vi "WPI_ADI_IMU_ComplementaryFilter.vi"(7 "Filter Coefficient a":dbl, 8 "dt (ms)":dbl, 10 "Gyro (degrees/second)":dbl, 11 "Accelerometer (degrees)":dbl) -> (2 "timeConstant":dbl, 3 "Filtered":dbl)   [LabVIEW 2015, in "FRC ADI MXP IMU.lvlib"]
uses:
  FRC ADI MXP IMU.lvlib
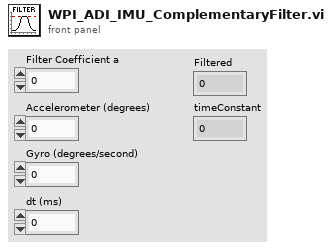
[diagram p1: front panel]
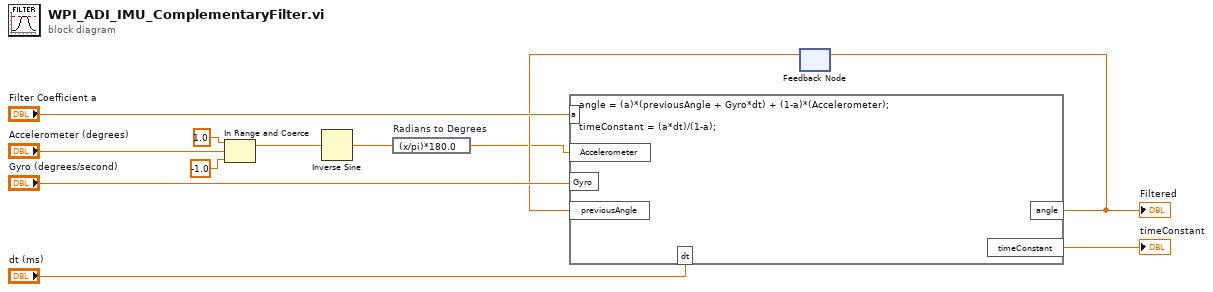
[diagram p0: block diagram]
diagram:
  n1 = In Range and Coerce(upper limit=1.0, x="Accelerometer (degrees)", lower limit=-1.0 ("upper limit")) -> (coerced(x)=w5:dbl)  [unwired: 1 out]
  n2 = Inverse Sine(1:w5) -> (0:w6:dbl)
  n3 = expression code="(x/pi)*180.0" "Radians to Degrees"(w6) -> (w1:dbl)
  n4 = feedback #1() -> (w7:dbl)  [unwired: 1 in]
  n5 = formula code="angle = (a)*(previousAngle + Gyro*dt) + (1-a)*(Accelerometer);\n\ntimeConstant = (a*dt)/(1-a);"("a"="Filter Coefficient a", "previousAngle"=w7, "dt"="dt (ms)", "Accelerometer"=w1, "Gyro"="Gyro (degrees/second)") -> ("angle"=w8:dbl, "timeConstant"=→"timeConstant":dbl)
  "Filtered" <- w8
  n6 = feedback-in #1(w8) -> ()
